vi "IRSensorReadBug.vi"(2 "NXT 2":T4={"Hardware"="NXT", "Flattened String"=""}, 3 "Port/MUX":T2 {"Port" items=["Port 1", "Port 2", "Port 3", "Port 4"]; "MUX Port" items=["No MUX", "MUX 1", "MUX 2", "MUX 3", "MUX 4"]}) -> (1 "All Info":T1, 4 "NXT":T4={"Hardware"="NXT", "Flattened String"=""})   [LabVIEW 2010]
uses:
  <vilib>/NXT/Subs/LVHSConnector.ctl
  <vilib>/NXT/HiTechnic/HiTechnic Controls/HiTechnic Port.ctl
  <vilib>/NXT/Block Support/NXT_InputPort.ctl
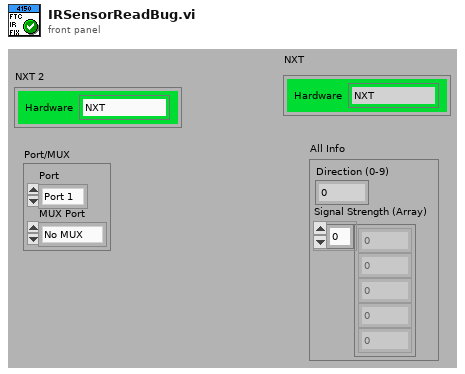
[diagram p1: front panel]
types:
  T1 = cluster{"Direction (0-9)":i16, "Signal Strength (Array)":u8[]}
  T2 = typedef "HiTechnic Port.ctl" = cluster{"Port":T3, "MUX Port":u8}
  T3 = typedef "NXT_InputPort.ctl" = u8
  T4 = typedef "LVHSConnector.ctl" = cluster{"Hardware":string, "Flattened String":string}
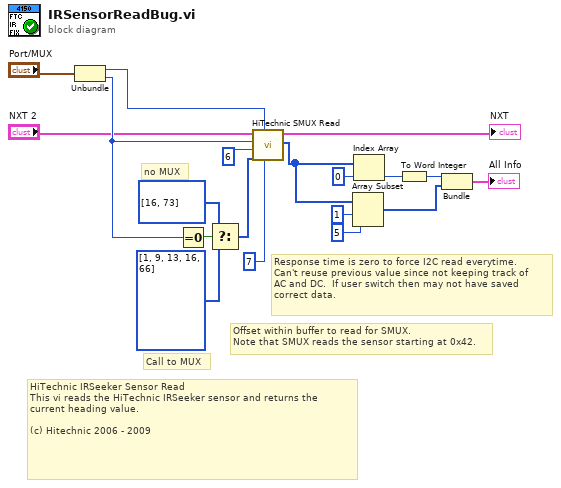
[diagram p0: block diagram]
diagram:
  # "Response time is zero to force I2C read everytime.\nCan't reuse previous value since not keeping track of\nAC and DC.  If user switch then may not have saved \ncorrect data."
  # "Offset within buffer to read for SMUX.  \nNote that SMUX reads the sensor starting at 0x42."
  # "no MUX"
  # "Call to MUX"
  # "HiTechnic IRSeeker Sensor Read\nThis vi reads the HiTechnic IRSeeker sensor and returns the\ncurrent heading value.  \n\n(c) Hitechnic 2006 - 2009"
  n1 = Unbundle("Port/MUX") -> ("Port"=w18:T3, "MUX Port"=w19:u8)
  n2 = Equal To 0?(x=w19) -> (x = 0?=w14:bool)
  n3 = Select(t=u8[] [16, 73] ("Buffer"), s=w14, f=u8[] [1, 9, 13, 16, 66]) -> (s? t:f=w17:u8[])
  n4 = call <vilib>:"HiTechnic SMUX Read.vi"("Offset"=u8 7, "Port"=w18, "Parameters"=w17, "Read Length"=u8 6, "MUX Port"=w19, "NXT"="NXT 2") -> ("Array"=w4:u8[], "NXT"=→"NXT":T4)  [unwired: 4 in]
  n5 = Array Subset(array=w4, index=1, length=5) -> (w5:u8[])
  n6 = Index Array(array=w4, index=0) -> (element=w2:u8)
  n7 = To Word Integer(number=w2) -> (16bit integer=w3:i16)
  n8 = Bundle(w3, w5) -> (→"All Info":cluster{i16, u8[]})  [unwired: 1 in]
